vi "GetAllTreeItems.vi"(11 "Tree In":refnum<data-value>) -> (3 "Tree Out":refnum<data-value>)   [LabVIEW 2019]
uses:
  Tree.lvclass
panel:
  out "Names":string[](array[string])
  out "Nodes Out":variant[](array[variant])
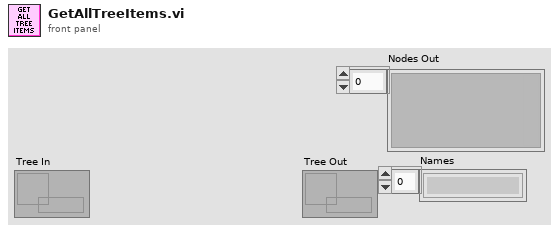
[diagram p1: front panel]
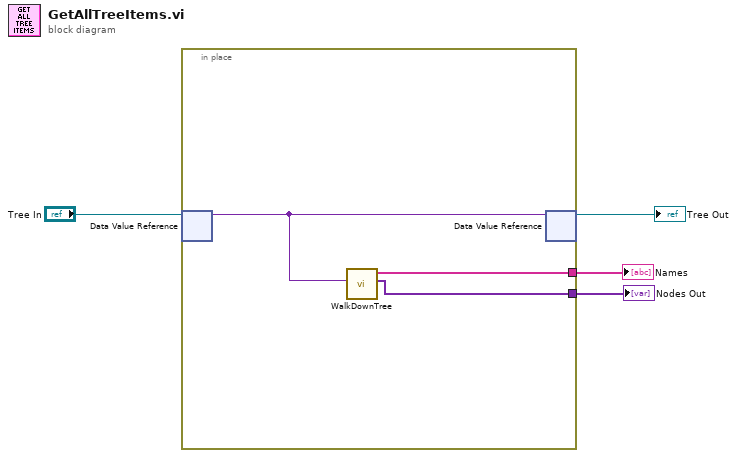
[diagram p0: block diagram]
diagram:
  n1 = in-place {
    in-place-border: [w6] -> w2
    in-place-border: [w5] -> w1
    n2 = in-place-dvr #1("Tree In") -> (w7:variant)  [unwired: 1 out]
    n3 = call "WalkDownTree.vi"("Node In"=w7) -> ("Nodes Out"=w5:variant[], "Names"=w6:string[])  [unwired: 8 in, 1 out]
    n4 = in-place-dvr #1(w7) -> (→"Tree Out":refnum<data-value>)  [unwired: 1 out]
  }
  "Names" <- w2
  "Nodes Out" <- w1
